vi "ServoCommunication_Initialization.vi"() -> ()   [LabVIEW 2024]
uses:
  DataTypes/ServoConnectionParameters.ctl
  DataTypes/OperationTypeForFunctionalGlobalVariable.ctl
  <vilib>/Utility/config.llb/Read Key (String).vi
  <vilib>/Utility/config.llb/Read Key (U32).vi
  <vilib>/Utility/config.llb/Read Key (Boolean).vi
  <vilib>/Utility/config.llb/NI_LVConfig.lvlib
panel:
  out "base_url":string
  out "timeout_ms":u32
  out "use_https":bool
  out "port":u16
  out "host":string
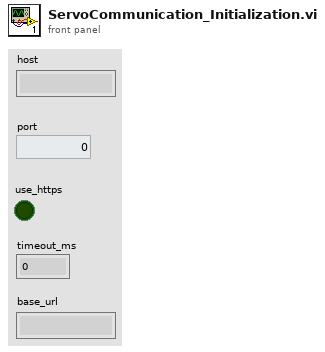
[diagram p1: front panel]
types:
  T1 = typedef "OperationTypeForFunctionalGlobalVariable.ctl" = enum16{"GET", "SET"}
  T2 = typedef "ServoConnectionParameters.ctl" = cluster{"host":string, "port":u16, "use_https":bool, "timeout_ms":u32, "base_url":string}
  T3 = typedef "NI_LVConfig.lvlib/Config Data RefNum.ctl" = refnum<k1>
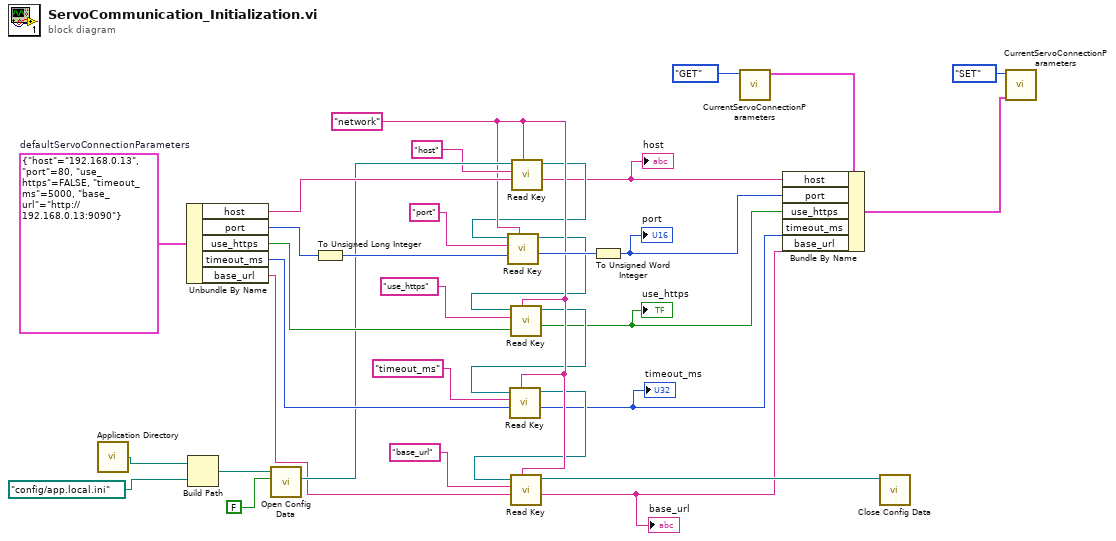
[diagram p0: block diagram]
diagram:
  w13 = "network" ("key")
  w27 = T2 {"host"="192.168.0.13", "port"=80, "use_https"=FALSE, "timeout_ms"=5000, "base_url"="http://192.168.0.13:9090"}  # defaultServoConnectionParameters
  n1 = call <vilib>:"Application Directory.vi"() -> ("Application Directory"=w7:path)
  n2 = Unbundle By Name(w27) -> ("host"=w26:string, "port"=w23:u16, "use_https"=w25:bool, "timeout_ms"=w24:u32, "base_url"=w14:string)
  n3 = Build Path(base path=w7, name or relative path=path "config/app.local.ini") -> (appended path=w6:path)
  n4 = call <vilib>:"Open Config Data.vi"("create file if necessary (T)"=FALSE, "configuration file path"=w6) -> ("refnum"=w21:T3)  [unwired: 7 in, 2 out]
  n5 = To Unsigned Long Integer(number=w23) -> (unsigned 32bit integer=w22:u32)
  n6 = call-poly <vilib>:"Read Key.vi"("section"=w13, "default value"=w26, "key"="host", "refnum"=w21) -> ("value"=w5:string, "refnum out"=w11:T3)  [unwired: 4 in, 2 out]
  "host" <- w5
  n7 = call-poly <vilib>:"Read Key.vi"("section"=w13, "default value"=w22, "key"="port", "refnum"=w11) -> ("value"=w20:u32, "refnum out"=w10:T3)  [unwired: 4 in, 2 out]
  n8 = call-poly <vilib>:"Read Key.vi"("section"=w13, "default value"=w25, "key"="use_https", "refnum"=w10) -> ("value"=w3:bool, "refnum out"=w9:T3)  [unwired: 4 in, 2 out]
  "use_https" <- w3
  n9 = call-poly <vilib>:"Read Key.vi"("section"=w13, "default value"=w24, "key"="timeout_ms", "refnum"=w9) -> ("value"=w2:u32, "refnum out"=w8:T3)  [unwired: 4 in, 2 out]
  "timeout_ms" <- w2
  n10 = call-poly <vilib>:"Read Key.vi"("section"=w13, "default value"=w14, "key"="base_url", "refnum"=w8) -> ("value"=w1:string, "refnum out"=w12:T3)  [unwired: 4 in, 2 out]
  "base_url" <- w1
  n11 = To Unsigned Word Integer(number=w20) -> (unsigned 16bit integer=w4:u16)
  "port" <- w4
  n12 = call "CurrentServoConnectionParameters.vi"("Operation"=OperationTypeForFunctionalGlobalVariable."GET") -> ("Current Servo Connection Parameters"=w29:T2)  [unwired: 10 in]
  n13 = Bundle By Name(cluster=w29, "host"=w5, "port"=w4, "use_https"=w3, "timeout_ms"=w2, "base_url"=w1) -> (w28:T2)
  n14 = call <vilib>:"Close Config Data.vi"("refnum"=w12) -> ()  [unwired: 9 in, 2 out]
  n15 = call "CurrentServoConnectionParameters.vi"("New Servo Connection Parameters"=w28, "Operation"=OperationTypeForFunctionalGlobalVariable."SET") -> ()  [unwired: 9 in, 1 out]
